vi "이벤트핸들러.vi"() -> ()   [LabVIEW 2014]
uses:
  <vilib>/Analysis/NI_AALBase.lvlib
panel:
  in  "정지":bool
  in  "삼각파형":bool
  in  "사인파형":bool
  out "웨이브폼 그래프":dbl[](graph)
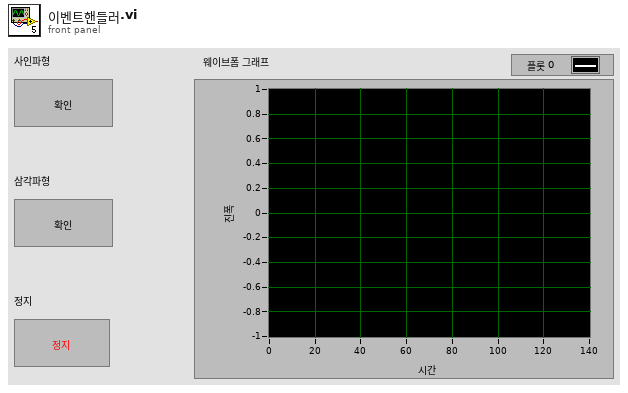
[diagram p1: front panel]
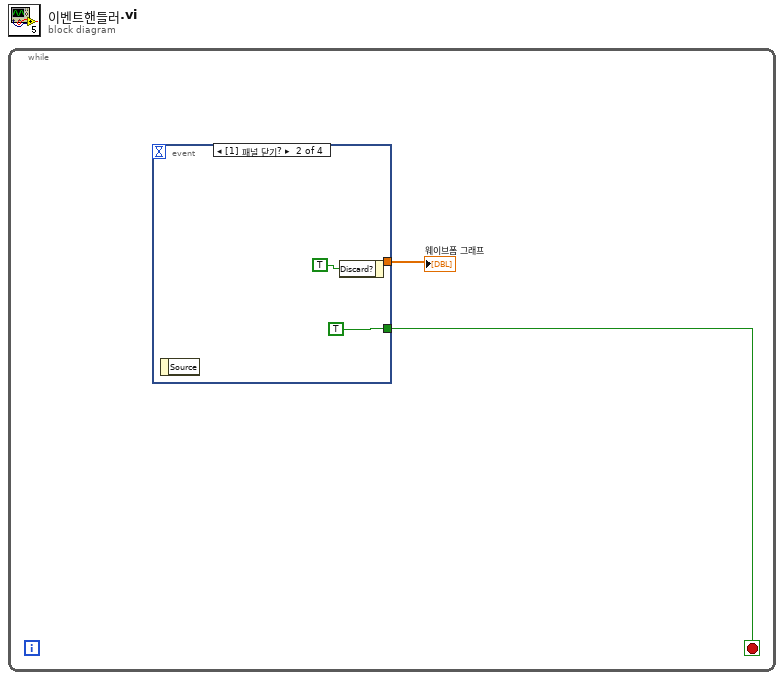
[diagram p0: block diagram]
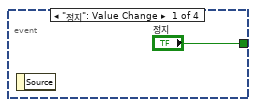
[diagram p2: hidden frame]
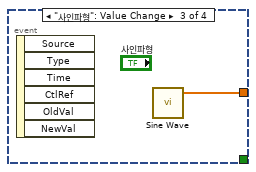
[diagram p3: hidden frame]
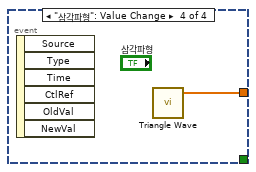
[diagram p4: hidden frame]
diagram:
  n1 = while {
    stop <- w2 stop-if-true
    n2 = event shown="[1] 패널 닫기?" {
      selector: _ -> [_ _ _ _]
      dyn-events: _ -> [_ _ _ _]
      timeout: _ -> [_ _ _ _]
      tunnel: ["정지" TRUE _ _] -> w2
      tunnel: [_ _ w6 w7] -> w1
      event "정지": Value Change {
        n3 = event-data() -> ()  [unwired: 1 in, 1 out]
      }
      event Panel Close? {
        n4 = event-data() -> ()  [unwired: 1 in, 1 out]
        n5 = event-data("Discard?"=TRUE) -> ()  [unwired: 1 in, 1 out]
      }
      event "사인파형": Value Change {
        n6 = event-data() -> ()  [unwired: 1 in, 6 out]
        n7 = call <vilib>:"Sine Wave.vi"() -> ("sine wave"=w6:dbl[])  [unwired: 5 in, 2 out]
      }
      event "삼각파형": Value Change {
        n8 = event-data() -> ()  [unwired: 1 in, 6 out]
        n9 = call <vilib>:"Triangle Wave.vi"() -> ("triangle wave"=w7:dbl[])  [unwired: 5 in, 2 out]
      }
    }
    "웨이브폼 그래프" <- w1
  }
